vi "read_data.vi"(8 "error in (no error)":errorcluster, 11 "LogisticRegression in":refnum<class "LogisticRegression.lvclass">) -> (0 "error out":errorcluster, 2 "data":T1, 3 "LogisticRegression out":refnum<class "LogisticRegression.lvclass">)   [LabVIEW 2020, in "LogisticRegression.lvclass"]
uses:
  LogisticRegression.lvclass
  Controls/logistic_regression_data.ctl
  LogisticRegression.lvclass/LogisticRegression.ctl
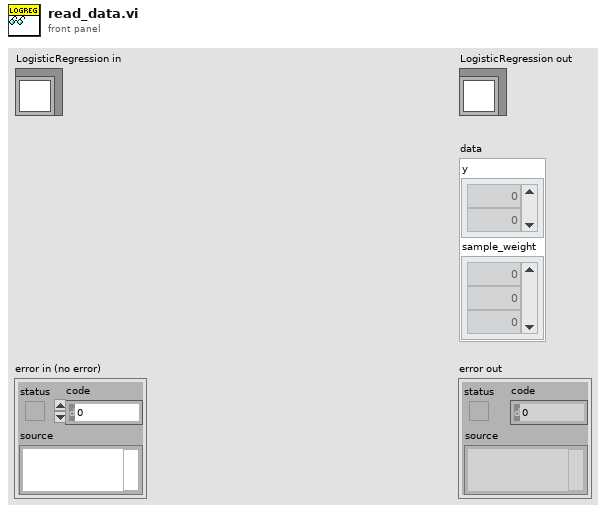
[diagram p1: front panel]
types:
  T1 = typedef "logistic_regression_data.ctl" = cluster{"y":dbl[], "sample_weight":dbl[]}
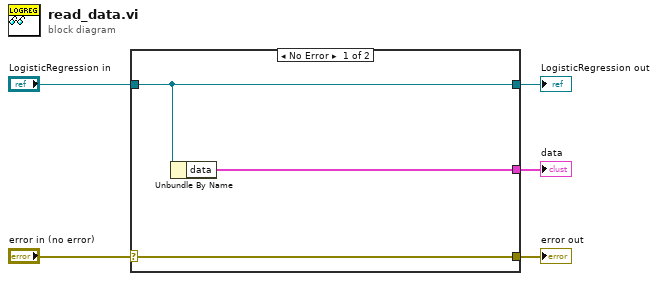
[diagram p0: block diagram]
diagram:
  n1 = case shown="No Error" "error in (no error)" {
    selector: "error in (no error)" -> [w8 w9]
    tunnel: [w8 w9] -> w4
    tunnel: [w7 w10] -> w2
    tunnel: "LogisticRegression in" -> [w7 w10]
    tunnel: [w6 _] -> w1
    frame No Error {
      n2 = Unbundle By Name(w7) -> ("data"=w6:T1)
    }
    frame Error {
    }
  }
  "error out" <- w4
  "LogisticRegression out" <- w2
  "data" <- w1
